vi "Write Error Logger's Enqueuer.vi"(8 "error in (no error)":errorcluster, 10 "Actor Framework:Message Enqueuer":refnum<class "Message Enqueuer.lvclass">, 11 "TCP_Listener in":refnum<class "TCP_Listener.lvclass">) -> (0 "error out":errorcluster, 3 "TCP_Listener out":refnum<class "TCP_Listener.lvclass">)   [LabVIEW 2023, in "TCP_Listener.lvlib" / "TCP_Listener.lvclass"]
uses:
  TCP_Listener.lvclass
  TCP_Listener.lvclass/TCP_Listener.ctl
  <vilib>/ActorFramework/Message Enqueuer/Message Enqueuer.lvclass
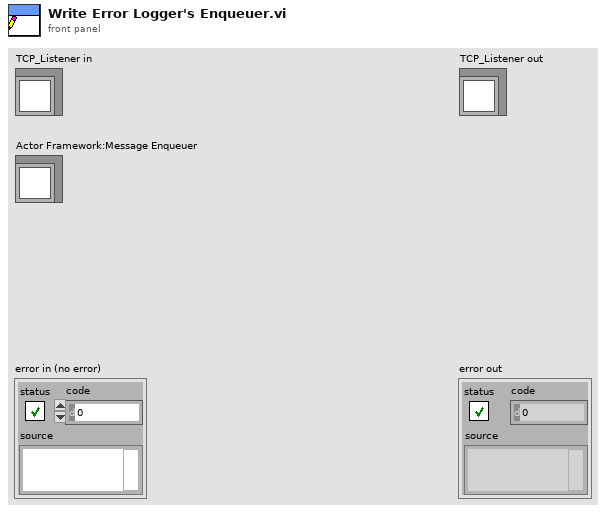
[diagram p1: front panel]
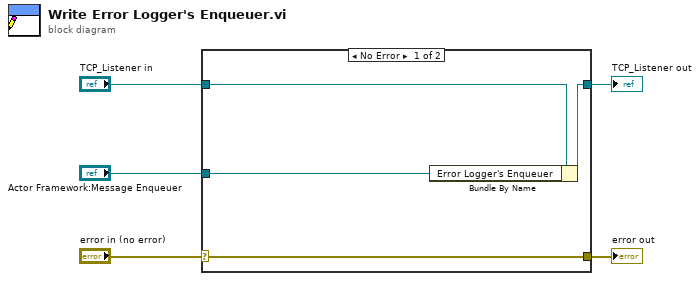
[diagram p0: block diagram]
diagram:
  n1 = case shown="No Error" "error in (no error)" {
    selector: "error in (no error)" -> [w9 w10]
    tunnel: [w9 w10] -> w4
    tunnel: [w7 w11] -> w2
    tunnel: "TCP_Listener in" -> [w8 w11]
    tunnel: "Actor Framework:Message Enqueuer" -> [w6 _]
    frame No Error {
      n2 = Bundle By Name(cluster=w8, "Error Logger's Enqueuer"=w6) -> (w7:refnum<class "TCP_Listener.lvclass">)
    }
    frame Error {
    }
  }
  "error out" <- w4
  "TCP_Listener out" <- w2
